vi "Formate Assertions for Description.vi"(10 "Item":string, 11 "Result Model in":refnum<class "Result Model.lvclass">) -> (2 "Assertions Description":string)   [LabVIEW 2020, in "Result Model.lvclass"]
uses:
  Result Model.lvclass
  Result Model.lvclass/Result Model.ctl
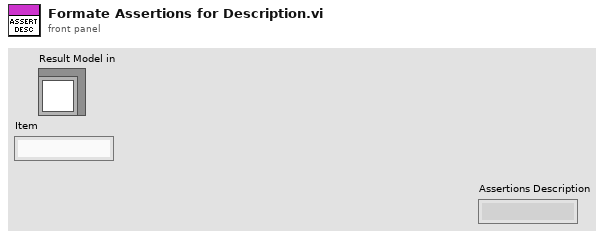
[diagram p1: front panel]
types:
  T1 = typedef "Result.lvlib/Type.ctl" = enum16{"Method", "Case", "Suite", "Pass", "Fail", "Skip", "Pass if", "Fail if", "Pass if Error", "Fail if Error", "Pass if Equal", "Fail if Equal"}
  T2 = typedef "Result.lvlib/Status.ctl" = enum16{"", "Passed", "Failed", "Error", "Skipped", "Setup Error", "Broken", "Teardown Error"}
  T3 = map{string, cluster{"Result Type":T1, "Status":T2, "Message":string, "Description":string}[]}
  T4 = cluster{"Result Type":T1, "Status":T2, "Message":string, "Description":string}[]
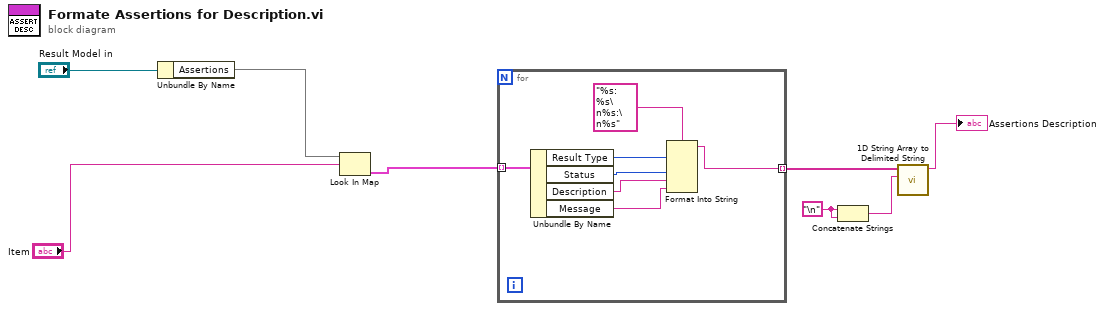
[diagram p0: block diagram]
diagram:
  w1 = "\n"
  n1 = Unbundle By Name("Result Model in") -> ("Assertions"=w7:T3)
  n2 = Look In Map(map=w7, key="Item") -> (value=w3:T4)  [unwired: 1 in, 1 out]
  n3 = for {
    tunnel: [w14] -> w6 mode=indexing
    tunnel: w3 -> [w11] mode=indexing
    n4 = Unbundle By Name(w11) -> ("Result Type"=w13:T1, "Status"=w12:T2, "Description"=w10:string, "Message"=w9:string)
    n5 = Format Into String(format string="%s: %s\n%s:\n%s", w13, w12, w10, w9) -> (resulting string=w14:string)  [unwired: 2 in, 1 out]
  }
  n6 = Concatenate Strings(w1, w1) -> (w2:string)
  n7 = call <vilib>:"1D String Array to Delimited String.vi"("delimiter"=w2, "string array"=w6) -> ("delimited string"=→"Assertions Description":string)  [unwired: 9 in]
